vi "current out.vi"(8 "error in":errorcluster caption="에러 입력", 9 "Current 배열":dbl[](array[numeric]), 11 "task/channels in":refnum<k21> caption="태스크/채널 입력") -> (0 "error out":errorcluster caption="에러 출력", 3 "task out":refnum<k21> caption="태스크 출력")   [LabVIEW 2013]
uses:
  <vilib>/DAQmx/write.llb/DAQmx Write (Analog 1D DBL NChan 1Samp).vi
  <vilib>/DAQmx/miscellaneous.llb/DAQmx Fill In Error Info.vi
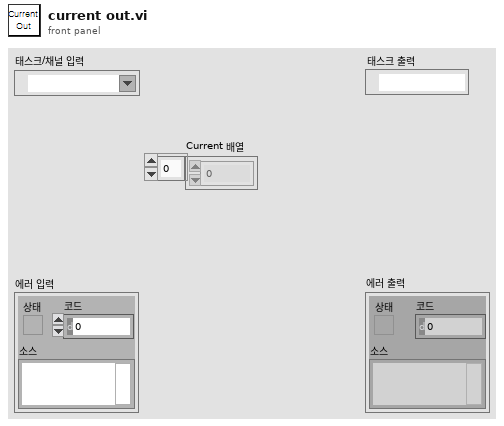
[diagram p1: front panel]
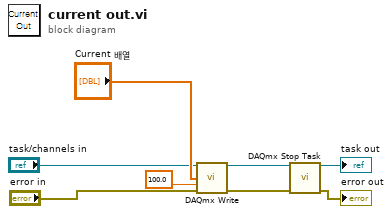
[diagram p0: block diagram]
diagram:
  n1 = call-poly <vilib>:"DAQmx Write.vi"("task/channels in"="task/channels in", "data"="Current 배열", "timeout"=100.0 ("timeout (s)"), "error in"="error in") -> ("task out"=w6:refnum<k21>, "error out"=w8:errorcluster)  [unwired: 9 in, 1 out]
  n2 = call <vilib>:"DAQmx Stop Task.vi"("task/channels in"=w6, "error in"=w8) -> ("task out"=→"task out":refnum<k21>, "error out"=→"error out":errorcluster)  [unwired: 12 in]
